vi "SubVI Open CLose.vi"() -> ()   [LabVIEW 2021]
panel:
  in  "stop":bool
  in  "Enum":enum16{"SubVI1", "SubVI2", "SubVI3"}(ring)
  in  "Go To Button":bool
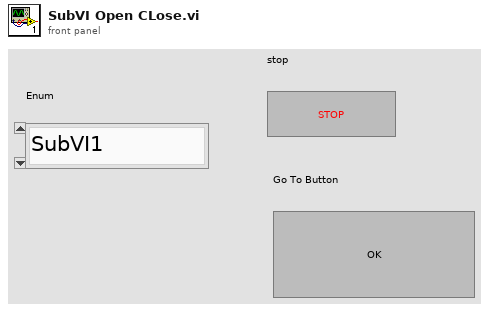
[diagram p1: front panel]
types:
  T1 = enum32{"Invalid", "Standard", "Closed", "Hidden", "Minimized", "Maximized"}
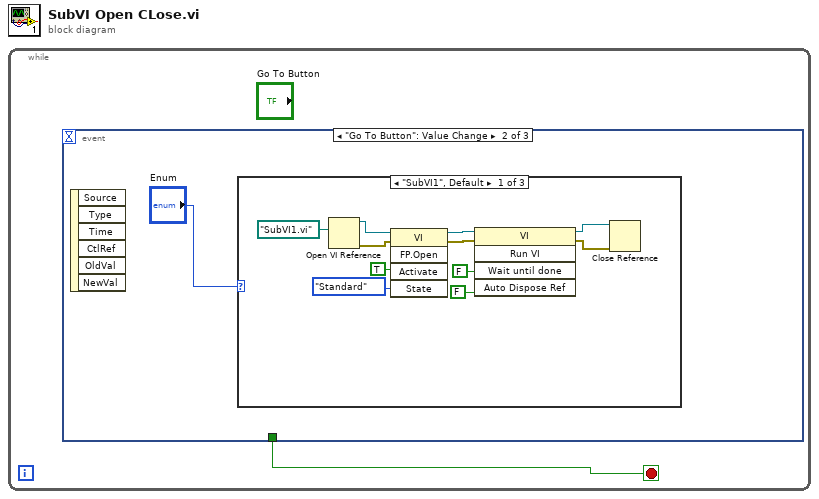
[diagram p0: block diagram]
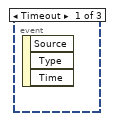
[diagram p2: hidden frame]
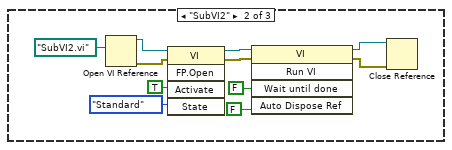
[diagram p3: hidden frame]
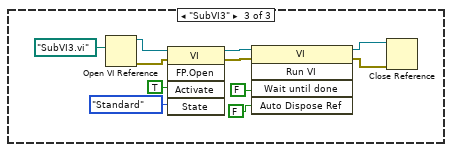
[diagram p4: hidden frame]
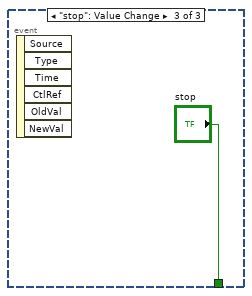
[diagram p5: hidden frame]
diagram:
  n1 = while {
    stop <- w1 stop-if-true
    n2 = event shown="[1] \"Go To Button\": Value Change" {
      selector: _ -> [_ _ _]
      dyn-events: _ -> [_ _ _]
      timeout: _ -> [_ _ _]
      tunnel: [_ _ "stop"] -> w1
      event Timeout {
        n3 = event-data() -> ()  [unwired: 1 in, 3 out]
      }
      event "Go To Button": Value Change {
        n4 = event-data() -> ()  [unwired: 1 in, 6 out]
        n5 = case shown="\"SubVI1\", Default" "Enum" {
          frame "SubVI1", Default {
            n6 = Open VI Reference(vi path=path "SubVI1.vi") -> (vi reference=w12:refnum<vi>, error out=w9:errorcluster)  [unwired: 5 in]
            n7 = invoke class="VI" method="FP.Open"(reference=w12, error in=w9, "Activate"=TRUE ("Activate?"), "State"=T1."Standard") -> (reference out=w8:refnum<vi>, error out=w7:errorcluster)  [unwired: 1 in, 3 out]
            n8 = invoke class="VI" method="Run VI"(reference=w8, error in=w7, "Wait until done"=FALSE, "Auto Dispose Ref"=FALSE) -> (reference out=w6:refnum<vi>, error out=w5:errorcluster)  [unwired: 1 in, 3 out]
            n9 = Close Reference(reference=w6, error in (no error)=w5) -> ()  [unwired: 1 out]
          }
          frame "SubVI2" {
            n10 = Open VI Reference(vi path=path "SubVI2.vi") -> (vi reference=w19:refnum<vi>, error out=w20:errorcluster)  [unwired: 5 in]
            n11 = invoke class="VI" method="FP.Open"(reference=w19, error in=w20, "Activate"=TRUE ("Activate?"), "State"=T1."Standard") -> (reference out=w21:refnum<vi>, error out=w22:errorcluster)  [unwired: 1 in, 3 out]
            n12 = invoke class="VI" method="Run VI"(reference=w21, error in=w22, "Wait until done"=FALSE, "Auto Dispose Ref"=FALSE) -> (reference out=w23:refnum<vi>, error out=w24:errorcluster)  [unwired: 1 in, 3 out]
            n13 = Close Reference(reference=w23, error in (no error)=w24) -> ()  [unwired: 1 out]
          }
          frame "SubVI3" {
            n14 = Open VI Reference(vi path=path "SubVI3.vi") -> (vi reference=w30:refnum<vi>, error out=w31:errorcluster)  [unwired: 5 in]
            n15 = invoke class="VI" method="FP.Open"(reference=w30, error in=w31, "Activate"=TRUE ("Activate?"), "State"=T1."Standard") -> (reference out=w32:refnum<vi>, error out=w33:errorcluster)  [unwired: 1 in, 3 out]
            n16 = invoke class="VI" method="Run VI"(reference=w32, error in=w33, "Wait until done"=FALSE, "Auto Dispose Ref"=FALSE) -> (reference out=w34:refnum<vi>, error out=w35:errorcluster)  [unwired: 1 in, 3 out]
            n17 = Close Reference(reference=w34, error in (no error)=w35) -> ()  [unwired: 1 out]
          }
        }
      }
      event "stop": Value Change {
        n18 = event-data() -> ()  [unwired: 1 in, 6 out]
      }
    }
  }
